vi "16-bit display mapping.vi"(8 "error in (no error)":errorcluster) -> (0 "error out":errorcluster)   [LabVIEW 2017]
uses:
  Globals/gl_Time series viewer globals.vi
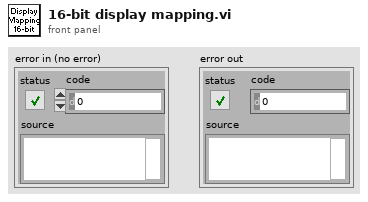
[diagram p1: front panel]
types:
  T1 = cluster{"Conversion Method":u32, "Minimum Value":i32, "Maximum Value":i32, "Number Of Shifts":i32}
  T2 = typedef "Time series viewer refs.ctl" = cluster{"This VI":refnum<vi>, "Image control":refnum<vi>, "AVI Mode ind":refnum<vi>, "Play":refnum<vi>, "Stop":refnum<vi>, "Back":refnum<vi>, "Scrollbar":refnum<vi>, "Video length info":refnum<vi>, "Expected speed values":refnum<vi>, "Intensity":refnum<vi>, "Path":refnum<vi>, "Selection sliders":refnum<vi>, "Speed Graph ref":refnum<vi>, "Frame rate set (fps)":refnum<vi>, "Channel to load":refnum<vi>, "Number of rows to generate":refnum<vi>, "Colour":refnum<vi>}
  T3 = typedef "Custom slider-horisontal.ctl" = cluster{dbl, dbl}
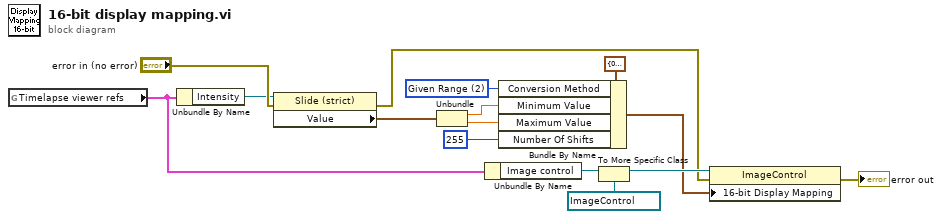
[diagram p0: block diagram]
diagram:
  w13 = u32 2 items=["Full Dynamic", "Downshift", "Given Range", "90% Dynamic", "Given Percent Range"] ("16-bit Display Mapping:Conversion Method")
  n1 = global read "gl_Time series viewer globals.vi" "Timelapse viewer refs"() -> (w5:T2)
  n2 = Unbundle By Name(w5) -> ("Intensity"=w8:refnum<vi>)
  n3 = property on="Property Node" class="Slide (strict)"(reference=w8, error in="error in (no error)") -> (error out=w1:errorcluster, "Value"=w14:T3)  [unwired: 1 out]
  n4 = Unbundle(w14) -> (w11:dbl, w12:dbl)
  n5 = Unbundle By Name(w5) -> ("Image control"=w6:refnum<vi>)
  n6 = Bundle By Name(cluster=T1 {"Conversion Method"=0, "Minimum Value"=0, "Maximum Value"=0, "Number Of Shifts"=0} ("16-bit Display Mapping:All Elements"), "Conversion Method"=w13, "Minimum Value"=w11, "Maximum Value"=w12, "Number Of Shifts"=255) -> (w3:T1)
  n7 = To More Specific Class(target class=refnum<vi> refnum ("Image"), reference=w6) -> (specific class reference=w4:refnum<vi>)  [unwired: 1 in, 1 out]
  n8 = property on="Property Node" class="ImageControl"(reference=w4, error in=w1, "16-bit Display Mapping"=w3) -> (error out=→"error out":errorcluster)  [unwired: 1 out]
